vi "Create Tree.vi"(8 "Error In":errorcluster, 10 "Eulogy Bookmarks":T1[](array[typedef]), 11 "TreeControl In":refnum<vi>) -> (0 "Error Out":errorcluster, 3 "TreeControl Out":refnum<vi>)   [LabVIEW 2017, in "Bookmark Manager.lvlib"]
uses:
  Bookmark Manager.lvlib
  VI Bookmark.ctl
  VI Information.ctl
  Application Information.ctl
  Eulogy/Public/Typedefs/Bookmarks.ctl
  Eulogy/Eulogy.lvlib
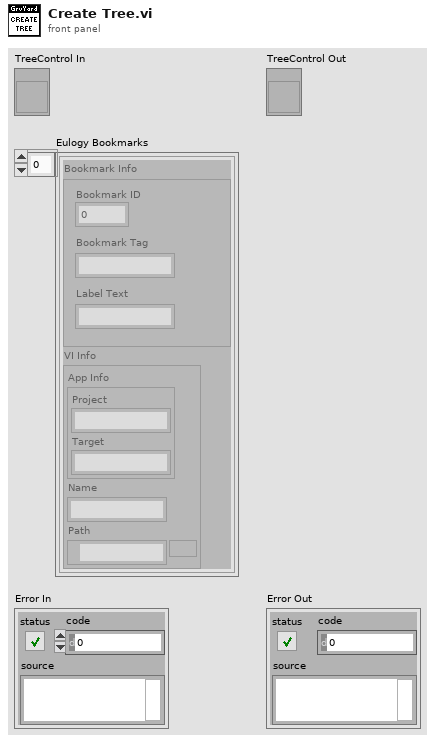
[diagram p1: front panel]
types:
  T1 = typedef "Bookmark Manager.lvlib/VI Bookmark.ctl" = cluster{"Bookmark Info":cluster{"Bookmark ID":u32, "Bookmark Tag":string, "Label Text":string}, "VI Info":T2}
  T2 = typedef "Bookmark Manager.lvlib/VI Information.ctl" = cluster{"App Info":T3, "Name":string, "Path":path}
  T3 = typedef "Bookmark Manager.lvlib/Application Information.ctl" = cluster{"Project":string, "Target":string}
  T4 = typedef "Eulogy.lvlib/Bookmarks.ctl" = enum16{"RIP", "Zombie"}
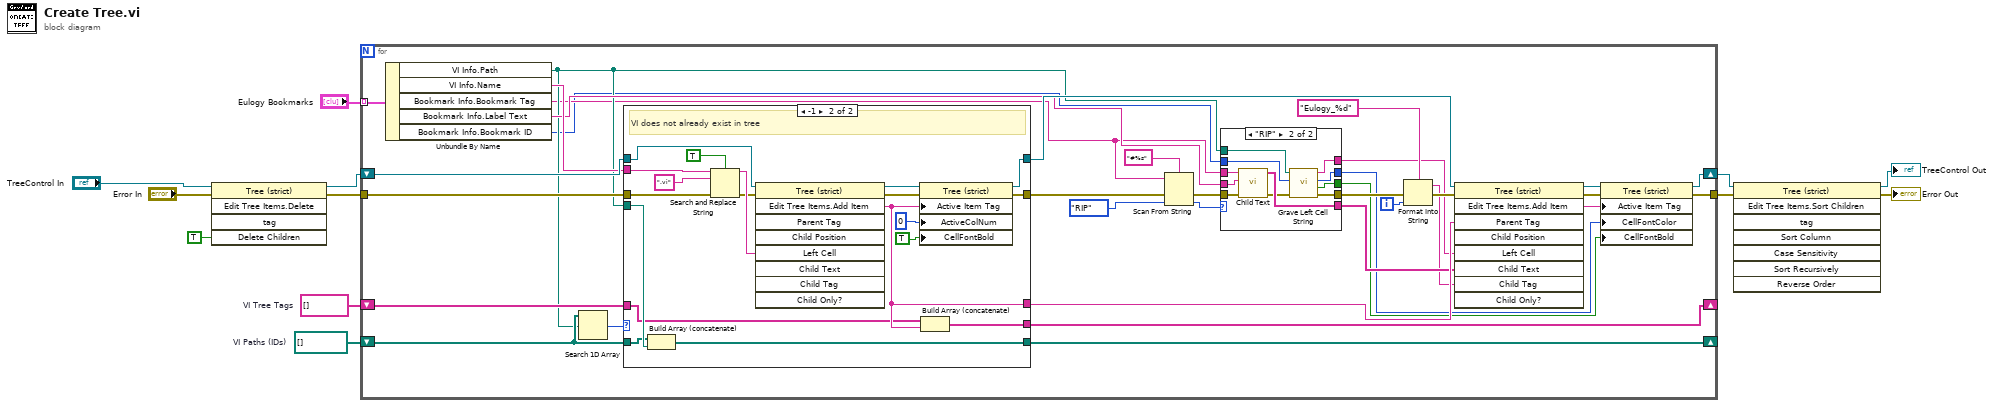
[diagram p0: block diagram]
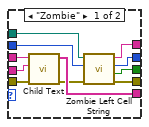
[diagram p2: hidden frame]
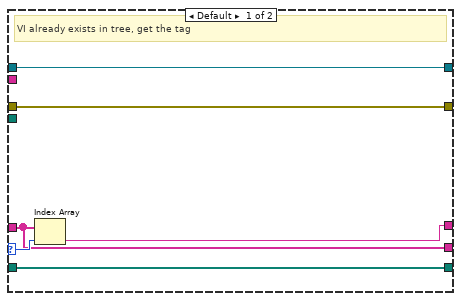
[diagram p3: hidden frame]
diagram:
  w1 = string[] []  # VI Tree Tags
  w2 = path[] []  # VI Paths (IDs)
  n1 = invoke class="Tree (strict)" method="Edit Tree Items.Delete"(reference="TreeControl In", error in="Error In", "Delete Children"=TRUE ("Delete Children?")) -> (reference out=w7:refnum<vi>, error out=w9:errorcluster)  [unwired: 2 in, 3 out]
  n2 = for {
    shift-right: [w19] -> w8
    shift-left: w7 -> [w45]
    tunnel: w9 -> [w46]
    tunnel: [w17] -> w11
    tunnel: "Eulogy Bookmarks" -> [w43] mode=indexing
    shift-right: [w39] -> _
    shift-left: w2 -> [w40]
    shift-right: [w38] -> _
    shift-left: w1 -> [w37]
    i -> [w21]
    n3 = Unbundle By Name(w43) -> ("VI Info.Path"=w30:path, "VI Info.Name"=w42:string, "Bookmark Info.Bookmark Tag"=w25:string, "Bookmark Info.Label Text"=w34:string, "Bookmark Info.Bookmark ID"=w24:u32)
    n4 = Search 1D Array(1D array=w40, element=w30) -> (index of element=w41:i32)  [unwired: 1 in]
    n5 = case shown="-1" w41 {
      selector: w41 -> [w73 _]
      tunnel: w46 -> [w70 w77]
      tunnel: w45 -> [w74 w93]
      tunnel: [w74 w91] -> w44
      tunnel: w42 -> [_ w80]
      tunnel: w30 -> [_ w87]
      tunnel: w40 -> [w69 w86]
      tunnel: [w69 w85] -> w39
      tunnel: [w71 w84] -> w35
      tunnel: [w72 w83] -> w38
      tunnel: w37 -> [w72 w82]
      tunnel: [w70 w81] -> w32
      frame Default {
        # "VI already exists in tree, get the tag"
        n6 = Index Array(array=w72, index=w73) -> (element=w71:string)
      }
      frame -1 {
        # "VI does not already exist in tree"
        n7 = Build Array (concatenate)(w86, w87) -> (w85:path[])
        n8 = Search and Replace String(case sensitive?=TRUE ("ignore case? (F)"), input string=w80, search string=".vi", error in=w77) -> (result string=w79:string, error out=w76:errorcluster)  [unwired: 4 in, 2 out]
        n9 = invoke class="Tree (strict)" method="Edit Tree Items.Add Item"(reference=w93, error in=w76, "Left Cell"=w79) -> (reference out=w92:refnum<vi>, error out=w90:errorcluster, "Edit Tree Items:Add Item"=w84:string)  [unwired: 6 in, 6 out]
        n10 = property class="Tree (strict)"(reference=w92, error in=w90, "Active Item Tag"=w84, "ActiveColNum"=0 ("Active Cell:Active Column Number"), "CellFontBold"=TRUE ("Active Cell:Cell Font:Bold")) -> (reference out=w91:refnum<vi>, error out=w81:errorcluster)
        n11 = Build Array (concatenate)(w82, w84) -> (w83:string[])
      }
    }
    n12 = Scan From String(format string="#%s", input string=w25, error in=w32, default 1=Bookmarks."RIP" ("Bookmark")) -> (error out=w29:errorcluster, output 1=w27:T4)  [unwired: 1 in, 2 out]
    n13 = case shown="\"RIP\"" w27 {
      tunnel: [w50 w61] -> w15
      tunnel: w34 -> [w56 w67]
      tunnel: [w55 w68] -> w33
      tunnel: w29 -> [w57 w66]
      tunnel: [w49 w60] -> w31
      tunnel: w30 -> [w52 w62]
      tunnel: w25 -> [w54 w65]
      tunnel: w24 -> [w51 w64]
      tunnel: [w48 w59] -> w14
      tunnel: [w47 w58] -> w13
      frame "Zombie" {
        # "Grave"
        n14 = call "Child Text.vi"("Error In"=w57, "Label Text"=w56, "Bookmark Tag"=w54) -> ("Error Out"=w53:errorcluster, "Child Text"=w55:string[])  [unwired: 7 in]
        n15 = call "Zombie Left Cell String.vi"("Error In"=w53, "Bookmark ID"=w51, "VI Path"=w52) -> ("Error Out"=w49:errorcluster, "Bold?"=w47:bool, "Color"=w48:u32, "Text"=w50:string)  [unwired: 5 in]
      }
      frame "RIP" {
        # "Zombie"
        n16 = call "Child Text.vi"("Error In"=w66, "Label Text"=w67, "Bookmark Tag"=w65) -> ("Error Out"=w63:errorcluster, "Child Text"=w68:string[])  [unwired: 7 in]
        n17 = call "Grave Left Cell String.vi"("Error In"=w63, "Bookmark ID"=w64, "VI Path"=w62) -> ("Error Out"=w60:errorcluster, "Bold?"=w58:bool, "Color"=w59:u32, "Text"=w61:string)  [unwired: 5 in]
      }
    }
    n18 = Format Into String(format string="Eulogy_%d", error in=w31, w21) -> (resulting string=w20:string, error out=w23:errorcluster)  [unwired: 1 in]
    n19 = invoke class="Tree (strict)" method="Edit Tree Items.Add Item"(reference=w44, error in=w23, "Parent Tag"=w35, "Left Cell"=w15, "Child Text"=w33, "Child Tag"=w20) -> (reference out=w36:refnum<vi>, error out=w18:errorcluster, "Edit Tree Items:Add Item"=w16:string)  [unwired: 3 in, 6 out]
    n20 = property class="Tree (strict)"(reference=w36, error in=w18, "Active Item Tag"=w16, "CellFontColor"=w14, "CellFontBold"=w13) -> (reference out=w19:refnum<vi>, error out=w17:errorcluster)
  }
  n21 = invoke class="Tree (strict)" method="Edit Tree Items.Sort Children"(reference=w8, error in=w11) -> (reference out=→"TreeControl Out":refnum<vi>, error out=→"Error Out":errorcluster)  [unwired: 6 in, 6 out]
